vi "MT_generate_signal.vi"(6 "duration (s)":dbl, 8 "error in":errorcluster, 9 "frequency (Hz)":dbl, 10 "amplitude":dbl, 11 "sampling rate (per second)":dbl) -> (0 "error out":errorcluster)   [LabVIEW 2019]
uses:
  <vilib>/Analysis/NI_AALPro.lvlib
panel:
  out "Waveform Graph":dynamicdata(graph)
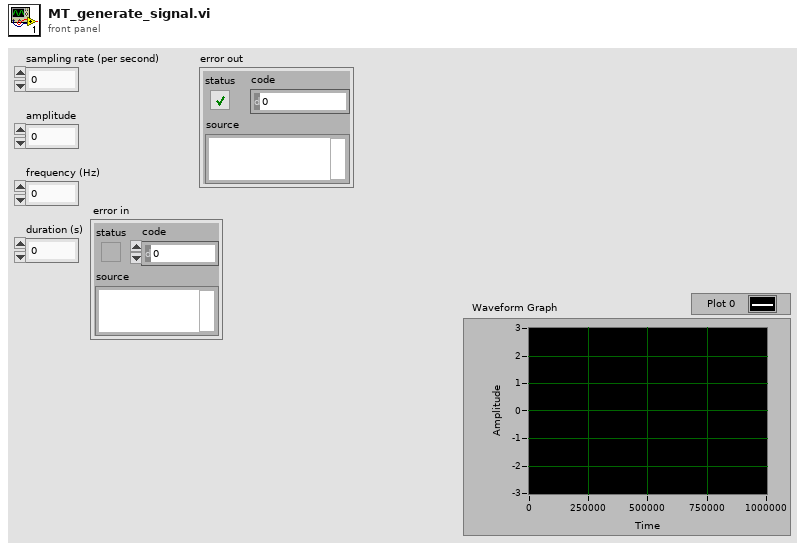
[diagram p1: front panel]
types:
  T1 = enum16{"sine", "cosine", "triangle", "square", "sawtooth", "increasing ramp", "decreasing ramp"}
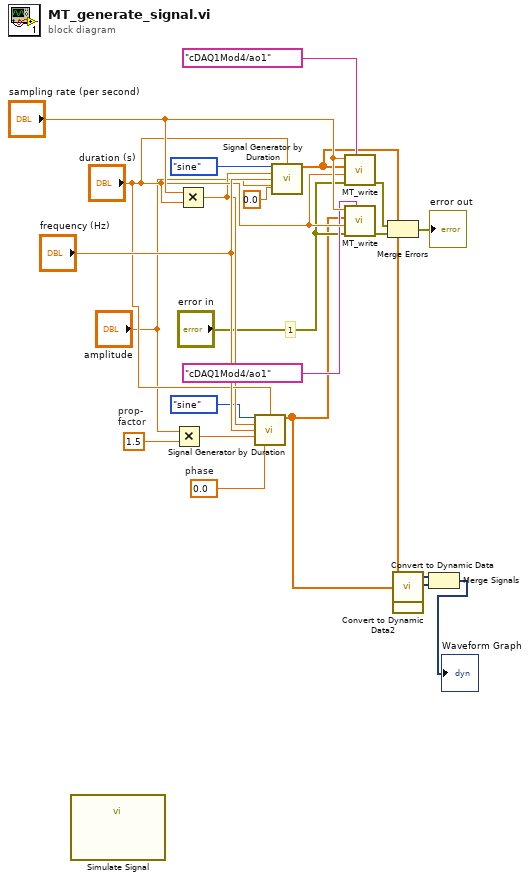
[diagram p0: block diagram]
diagram:
  w8 = 1.5  # prop- factor
  w10 = 0.0  # phase
  # "1"
  n1 = call "Simulate Signal"() -> ()  [unwired: 14 in, 2 out]
  n2 = Multiply(x="amplitude", y=w8) -> (x*y=w9:dbl)
  n3 = Multiply(x="sampling rate (per second)", y="duration (s)") -> (x*y=w15:dbl)
  n4 = call <vilib>:"Signal Generator by Duration.vi"("signal type"=T1."sine", "duration"="duration (s)", "# of samples"=w15, "frequency"="frequency (Hz)", "amplitude"=w9, "phase in"=w10) -> ("signal"=w3:dbl[])  [unwired: 6 in, 3 out]
  n5 = call <vilib>:"Signal Generator by Duration.vi"("signal type"=T1."sine", "duration"="duration (s)", "# of samples"=w15, "frequency"="frequency (Hz)", "amplitude"="amplitude", "phase in"=0.0) -> ("signal"=w5:dbl[])  [unwired: 6 in, 3 out]
  n6 = call "MT_write.vi"("Physical Channels"=tag "cDAQ1Mod4/ao1" ("Physical Channel"), "error in"="error in", "duration"="duration (s)", "signal"=w5, "sampling rate"="sampling rate (per second)") -> ("error out"=w18:errorcluster)  [unwired: 6 in]
  n7 = call "MT_write.vi"("Physical Channels"=tag "cDAQ1Mod4/ao1" ("Physical Channel"), "error in"="error in", "duration"="duration (s)", "signal"=w3, "sampling rate"="sampling rate (per second)") -> ("error out"=w19:errorcluster)  [unwired: 6 in]
  n8 = Merge Errors(w18, w19) -> (→"error out":errorcluster)
  n9 = call "Convert to Dynamic Data"("Array"=w5) -> ("Dynamic Data Type"=w4:dynamicdata)  [unwired: 3 in]
  n10 = call "Convert to Dynamic Data2"("Array"=w3) -> ("Dynamic Data Type"=w2:dynamicdata)  [unwired: 3 in]
  n11 = Merge Signals(w4, w2) -> (→"Waveform Graph":dynamicdata)
